vi "Homing_X_Stage.vi"() -> ()   [LabVIEW 2013]
panel:
  in  "MG17Motor":refnum<k7>(container)
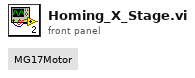
[diagram p1: front panel]
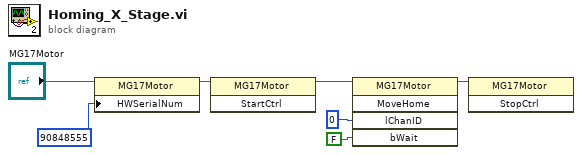
[diagram p0: block diagram]
diagram:
  n1 = property class="MG17Motor"(reference="MG17Motor", "HWSerialNum"=90848555) -> (reference out=w7:refnum<k7>)  [unwired: 1 in, 1 out]
  n2 = invoke class="MG17Motor" method="StartCtrl"(reference=w7) -> (reference out=w2:refnum<k7>)  [unwired: 2 in, 2 out]
  n3 = invoke class="MG17Motor" method="MoveHome"(reference=w2, "lChanID"=0, "bWait"=FALSE) -> (reference out=w5:refnum<k7>)  [unwired: 2 in, 4 out]
  n4 = invoke class="MG17Motor" method="StopCtrl"(reference=w5) -> ()  [unwired: 2 in, 3 out]
